vi "ElevatorNetworkSlowRead.vi"(8 "error in (no error)":errorcluster) -> (0 "error out":errorcluster)   [LabVIEW 2023]
uses:
  ElevatorGlobal.vi
  <vilib>/Rock Robotics/Network Tables/NT Write Number.vi
  <vilib>/Rock Robotics/Network Tables/NT Read Number.vi
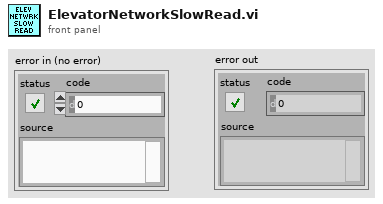
[diagram p1: front panel]
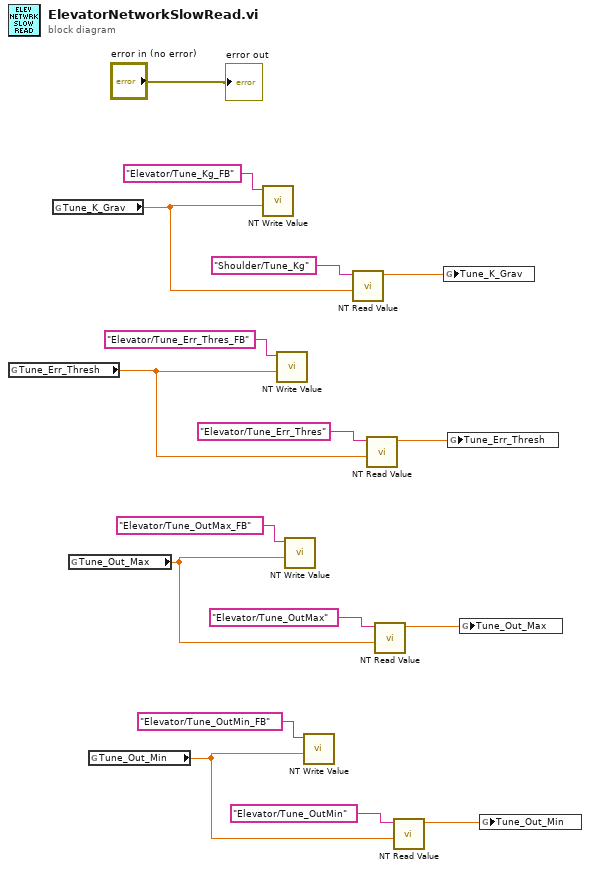
[diagram p0: block diagram]
diagram:
  n1 = global read "ElevatorGlobal.vi" "Tune_Err_Thresh"() -> (w9:dbl)
  n2 = global read "ElevatorGlobal.vi" "Tune_K_Grav"() -> (w13:dbl)
  n3 = global read "ElevatorGlobal.vi" "Tune_Out_Max"() -> (w5:dbl)
  n4 = global read "ElevatorGlobal.vi" "Tune_Out_Min"() -> (w1:dbl)
  n5 = call-poly <vilib>:"NT Write Value.vi"("value"=w13, "name"="Elevator/Tune_Kg_FB") -> ()  [unwired: 9 in, 1 out]
  n6 = call-poly <vilib>:"NT Write Value.vi"("value"=w9, "name"="Elevator/Tune_Err_Thres_FB") -> ()  [unwired: 9 in, 1 out]
  n7 = call-poly <vilib>:"NT Write Value.vi"("value"=w5, "name"="Elevator/Tune_OutMax_FB") -> ()  [unwired: 9 in, 1 out]
  n8 = call-poly <vilib>:"NT Write Value.vi"("value"=w1, "name"="Elevator/Tune_OutMin_FB") -> ()  [unwired: 9 in, 1 out]
  n9 = call-poly <vilib>:"NT Read Value.vi"("default value"=w13, "name"="Shoulder/Tune_Kg") -> ("value"=w14:dbl)  [unwired: 7 in, 2 out]
  n10 = call-poly <vilib>:"NT Read Value.vi"("default value"=w9, "name"="Elevator/Tune_Err_Thres") -> ("value"=w10:dbl)  [unwired: 7 in, 2 out]
  n11 = call-poly <vilib>:"NT Read Value.vi"("default value"=w5, "name"="Elevator/Tune_OutMax") -> ("value"=w6:dbl)  [unwired: 7 in, 2 out]
  n12 = call-poly <vilib>:"NT Read Value.vi"("default value"=w1, "name"="Elevator/Tune_OutMin") -> ("value"=w2:dbl)  [unwired: 7 in, 2 out]
  n13 = global write "ElevatorGlobal.vi" "Tune_K_Grav"(w14) -> ()
  n14 = global write "ElevatorGlobal.vi" "Tune_Err_Thresh"(w10) -> ()
  n15 = global write "ElevatorGlobal.vi" "Tune_Out_Max"(w6) -> ()
  n16 = global write "ElevatorGlobal.vi" "Tune_Out_Min"(w2) -> ()
  "error out" <- "error in (no error)"
